vi "Create From Variant (Object).vi"(8 "error in (no error)":errorcluster, 10 "Variant":variant) -> (0 "error out":errorcluster, 3 "JSON Value out":refnum<class "JSON Value.lvclass">)   [LabVIEW 2016, in "JSFL Variant Support.lvlib"]
doc: "Creates a new JSON instance from the given Variant."
uses:
  JSFL Variant Support.lvlib
  JSON Value.lvclass
  New JSON Value/New JSON ({Value[]}).vi
  <vilib>/Utility/Data Type/NI_Data Type.lvlib
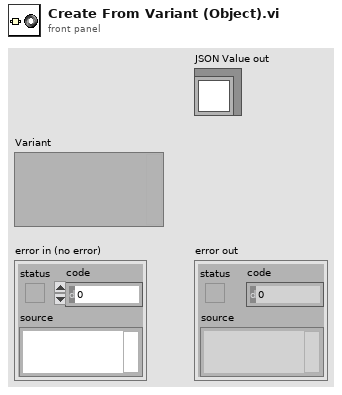
[diagram p1: front panel]
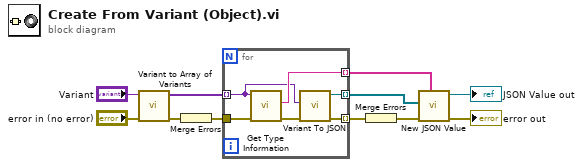
[diagram p0: block diagram]
diagram:
  n1 = call "Variant to Array of Variants.vi"("error in (no error)"="error in (no error)", "variant"="Variant") -> ("error out"=w2:errorcluster, "Array"=w3:variant[])  [unwired: 8 in]
  n2 = Merge Errors(w2) -> (w11:errorcluster)
  n3 = for {
    tunnel: w3 -> [w15] mode=indexing
    tunnel: [w14] -> w5 mode=indexing
    tunnel: [w17] -> w6 mode=indexing
    tunnel: w11 -> [w16]
    tunnel: [w13] -> w10 mode=indexing
    n4 = call <vilib>:"Get Type Information.vi"("error in (no error)"=w16, "Variant"=w15) -> ("error out"=w12:errorcluster, "Name"=w17:string)  [unwired: 5 in, 3 out]
    n5 = call "Variant To JSON.vi"("error in (no error)"=w12, "Variant"=w15) -> ("error out"=w13:errorcluster, "JSON Value out"=w14:refnum<class "JSON Value.lvclass">)  [unwired: 8 in]
  }
  n6 = Merge Errors(w10) -> (w9:errorcluster)
  n7 = call-poly "New JSON Value.vi"("keys"=w6, "error in (no error)"=w9, "values"=w5) -> ("error out"=→"error out":errorcluster, "JSON Value out"=→"JSON Value out":refnum<class "JSON Value.lvclass">)  [unwired: 7 in]
